vi "Construct Viewable Launches Dialog Box.vi"(10 "DialogBox to Launch":refnum<class "IDialogBox.lvclass">) -> (3 "ViewableLaunchesDialogBox":refnum<class "ViewableLaunchesDialogBox.lvclass">)   [LabVIEW 2020, in "ViewableLaunchesDialogBox.lvclass"]
uses:
  ViewableLaunchesDialogBox.lvclass
  Source/IDialogBox/IDialogBox/IDialogBox.lvclass
  ViewableLaunchesDialogBox.lvclass/ViewableLaunchesDialogBox.ctl
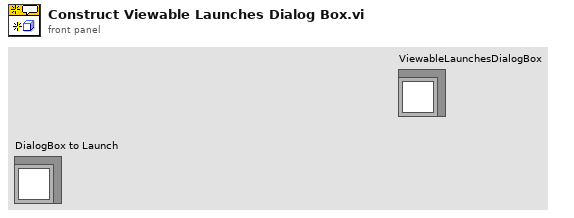
[diagram p1: front panel]
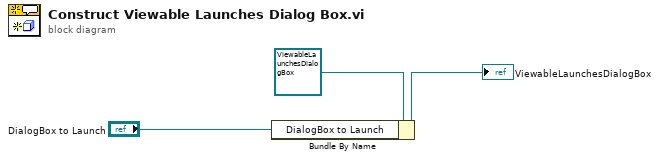
[diagram p0: block diagram]
diagram:
  n1 = Bundle By Name(cluster=refnum<class "ViewableLaunchesDialogBox.lvclass"> refnum ("ViewableLaunchesDialogBox in"), "DialogBox to Launch"="DialogBox to Launch") -> (→"ViewableLaunchesDialogBox":refnum<class "ViewableLaunchesDialogBox.lvclass">)
